vi "Status Msg Joiner.vi"(1 "History":string, 2 "Status Messages":string, 3 "Add?":bool=TRUE) -> (0 "Status Out":string)   [LabVIEW 2012]
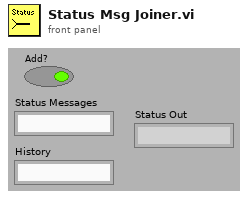
[diagram p1: front panel]
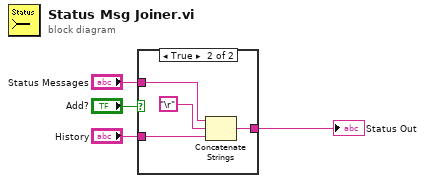
[diagram p0: block diagram]
diagram:
  n1 = case shown="True" "Add?" {
    tunnel: [w5 w9] -> w4
    tunnel: "History" -> [w5 w8]
    tunnel: "Status Messages" -> [_ w7]
    frame False {
    }
    frame True {
      n2 = Concatenate Strings(w7, "\r", w8) -> (w9:string)
    }
  }
  "Status Out" <- w4
